vi "Устройство вывода.vi"(4 "F":T3, 5 "read":bool, 6 "c":bool, 7 "A":T4) -> (0 "flags":T2, 1 "dig1":T1, 2 "dig0":T1, 3 "sign":bool)   [LabVIEW 2013]
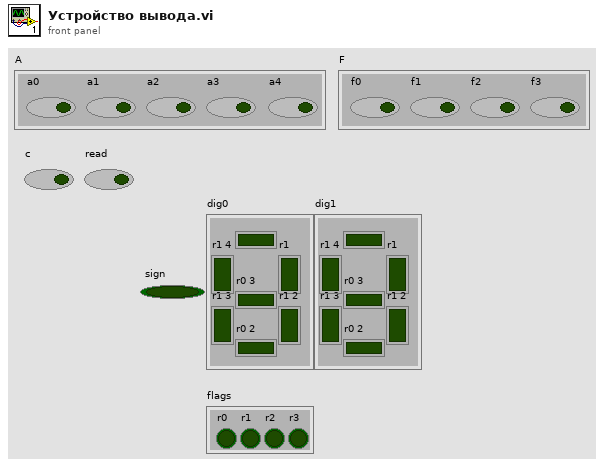
[diagram p1: front panel]
types:
  T1 = cluster{"r0":bool, "r1":bool, "r1 2":bool, "r0 2":bool, "r1 3":bool, "r1 4":bool, "r0 3":bool}
  T2 = cluster{"r0":bool, "r1":bool, "r2":bool, "r3":bool}
  T3 = cluster{"f0":bool, "f1":bool, "f2":bool, "f3":bool}
  T4 = cluster{"a0":bool, "a1":bool, "a2":bool, "a3":bool, "a4":bool}
  T5 = cluster{"q4":bool, "q3":bool, "q2":bool, "q1":bool, "q0":bool}
  T6 = cluster{"q3":bool, "q2":bool, "q1":bool, "q0":bool}
  T7 = cluster{"a":bool, "b":bool, "c":bool, "d":bool, "e":bool, "f":bool, "g":bool}
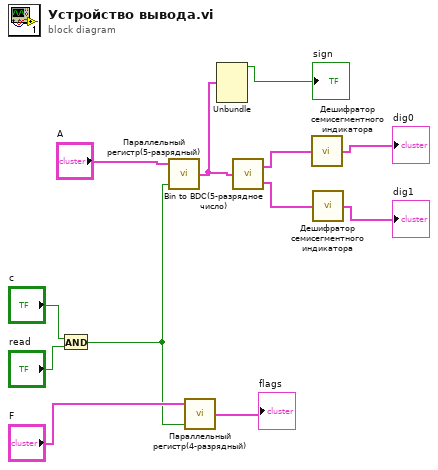
[diagram p0: block diagram]
diagram:
  n1 = And(x="c", y="read") -> (x .and. y?=w6:bool)
  n2 = call "Параллельный регистр(5-разрядный).vi"("C"=w6, "Cluster"="A") -> ("output cluster"=w3:T5)  [unwired: 1 in]
  n3 = call "Параллельный регистр(4-разрядный).vi"("C"=w6, "Cluster"="F") -> ("output cluster"=→"flags":T6)  [unwired: 1 in]
  n4 = Unbundle(w3) -> ("q4"=→"sign":bool)  [unwired: 4 out]
  n5 = call "Bin to BDC(5-разрядное число).vi"("B"=w3) -> ("R0"=w2:T2, "R1"=w1:T2)
  n6 = call "Дешифратор семисегментного индикатора.vi"("X"=w2) -> ("R"=→"dig0":T7)
  n7 = call "Дешифратор семисегментного индикатора.vi"("X"=w1) -> ("R"=→"dig1":T7)
